vi "TCP_Client.vi"() -> ()   [LabVIEW 2020]
panel:
  out "data out":string
  in  "stop":bool
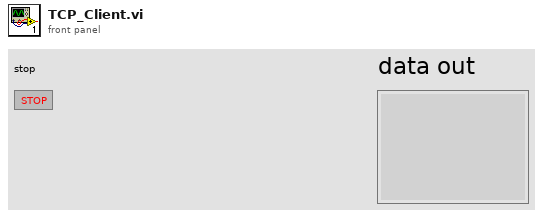
[diagram p1: front panel]
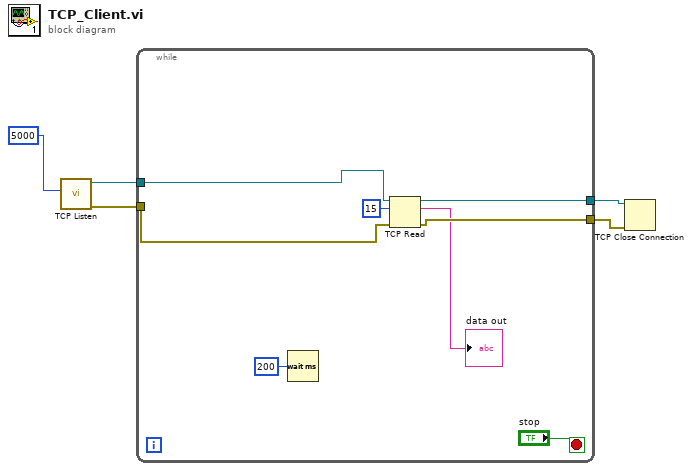
[diagram p0: block diagram]
diagram:
  n1 = call <vilib>:"TCP Listen.vi"("port"=u16 5000) -> ("error out"=w3:errorcluster, "connection ID"=w4:refnum<k5>)  [unwired: 6 in, 3 out]
  n2 = while {
    tunnel: w4 -> [w12]
    tunnel: w3 -> [w11]
    tunnel: [w9] -> w2
    tunnel: [w8] -> w1
    stop <- "stop" stop-if-true
    n3 = Wait (ms)(milliseconds to wait=u32 200) -> ()  [unwired: 1 out]
    n4 = TCP Read(connection ID=w12, bytes to read=15, error in (no error)=w11) -> (connection ID out=w9:refnum<k5>, data out=→"data out":string, error out=w8:errorcluster)  [unwired: 2 in]
  }
  n5 = TCP Close Connection(connection ID=w2, error in (no error)=w1) -> ()  [unwired: 1 in, 2 out]
